vi "Read XML_Parse Read Data.vi"(6 "Close Ref?":bool=TRUE, 8 "error in (no error)":errorcluster, 11 ".NET Refnum in":refnum<k24>) -> (0 "error out":errorcluster, 2 ".NET Refnum out":refnum<k24>, 3 "Channels":T1[](array[typedef]))   [LabVIEW 2017]
uses:
  XML_Channel.ctl
  XML_Label.ctl
  XML_Parameter.ctl
  D:/Ballard-Arinc-429-Custom-Device/Source/System Explorer/SubVIs/Parse Parameters File/Parameters_Arinc429_XML_Tools.dll
  Ballard-Arinc-429-Custom-Device/Source/System Explorer/SubVIs/Parse Parameters File/Parameters_Arinc429_XML_Tools.dll
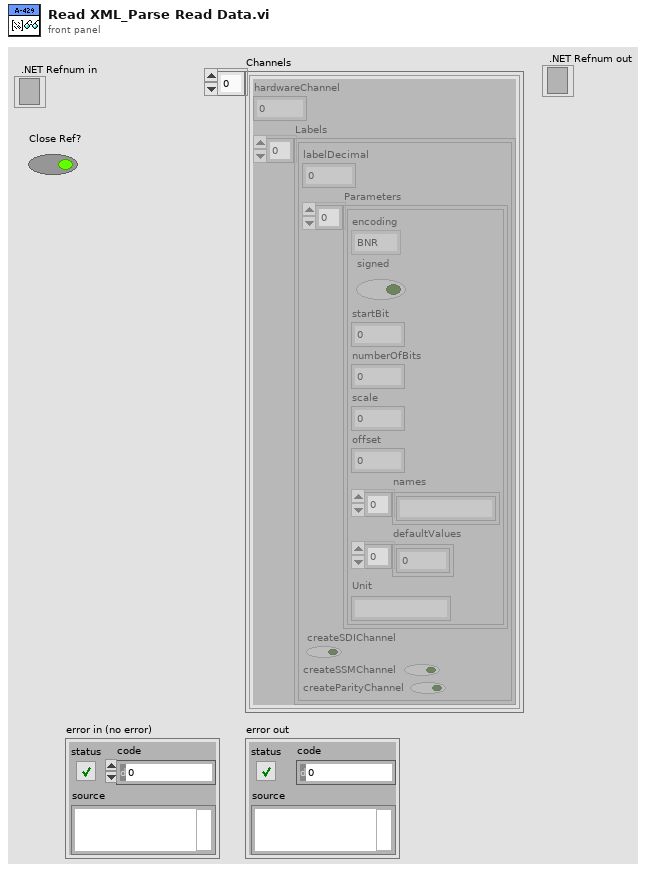
[diagram p1: front panel]
types:
  T1 = typedef "XML_Channel.ctl" = cluster{"hardwareChannel":i32, "Labels":T2[]}
  T2 = typedef "XML_Label.ctl" = cluster{"labelDecimal":i32, "Parameters":T3[], "createSDIChannel":bool, "createSSMChannel":bool, "createParityChannel":bool}
  T3 = typedef "XML_Parameter.ctl" = cluster{"encoding":enum16{"BNR", "BCD", "Discrete"}, "signed":bool, "startBit":i32, "numberOfBits":i32, "scale":dbl, "offset":dbl, "names":string[], "defaultValues":dbl[], "Unit":string}
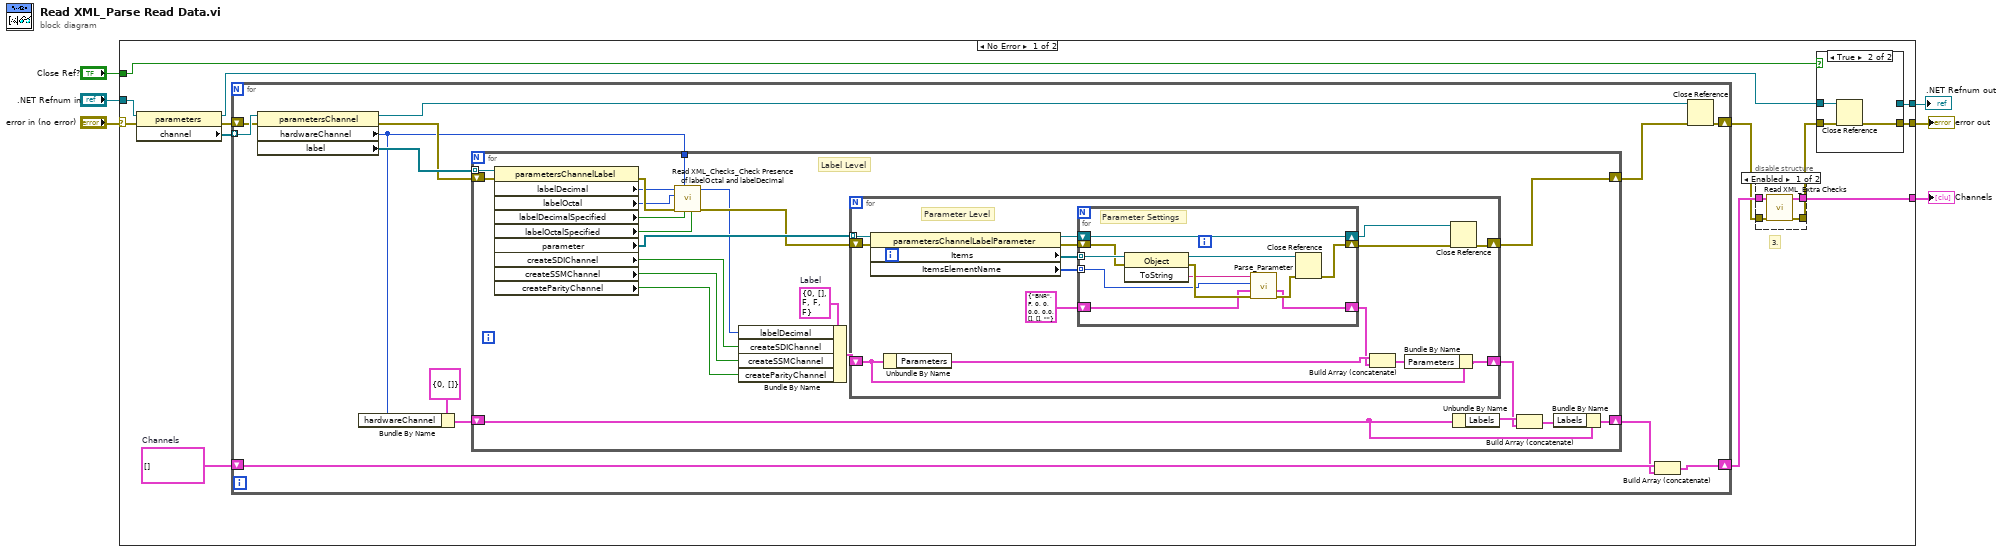
[diagram p0: block diagram]
diagram:
  n1 = case shown="No Error" "error in (no error)" {
    selector: "error in (no error)" -> [w9 w92]
    tunnel: [w17 _] -> w6
    tunnel: ".NET Refnum in" -> [w11 _]
    tunnel: [w10 w92] -> w4
    tunnel: "Close Ref?" -> [w8 _]
    tunnel: [w7 _] -> w1
    frame No Error {
      w18 = T1[] []  # Channels
      # "3."
      n2 = property class="parameters"(reference=w11, error in=w9) -> (reference out=w13:refnum<k24>, error out=w14:errorcluster, "channel"=w12:refnum<k24>[])
      n3 = for {
        tunnel: w12 -> [w43] mode=indexing
        shift-right: [w40] -> w15
        shift-left: w14 -> [w42]
        shift-right: [w33] -> w19
        shift-left: w18 -> [w34]
        n4 = property class="parametersChannel"(reference=w43, error in=w42) -> (reference out=w41:refnum<k24>, error out=w38:errorcluster, "hardwareChannel"=w31:i32, "label"=w39:refnum<k24>[])
        n5 = Bundle By Name(cluster=T1 {"hardwareChannel"=0, "Labels"=[]} ("Channel"), "hardwareChannel"=w31) -> (w35:T1)
        n6 = for {
          tunnel: w39 -> [w65] mode=indexing
          shift-right: [w62] -> w37
          shift-left: w38 -> [w64]
          shift-right: [w55] -> w32
          shift-left: w35 -> [w57]
          tunnel: w31 -> [w44]
          w61 = T2 {"labelDecimal"=0, "Parameters"=[], "createSDIChannel"=FALSE, "createSSMChannel"=FALSE, "createParityChannel"=FALSE}  # Label
          # "Label Level"
          n7 = property class="parametersChannelLabel"(reference=w65, error in=w64) -> (error out=w51:errorcluster, "labelDecimal"=w48:i32, "labelOctal"=w47:i32, "labelDecimalSpecified"=w46:bool, "labelOctalSpecified"=w45:bool, "parameter"=w63:refnum<k24>[], "createSDIChannel"=w54:bool, "createSSMChannel"=w53:bool, "createParityChannel"=w52:bool)  [unwired: 1 out]
          n8 = call "Read XML_Checks_Check Presence of labelOctal and labelDecimal.vi"("labelOctalSpecified"=w45, "labelDecimalSpecified"=w46, "hardwareChannel"=w44, "error in (no error)"=w51, "labelOctal"=w47, "labelDecimal"=w48) -> ("error out"=w50:errorcluster, "labelDecimal"=w49:i32)  [unwired: 4 in]
          n9 = Bundle By Name(cluster=w61, "labelDecimal"=w49, "createSDIChannel"=w54, "createSSMChannel"=w53, "createParityChannel"=w52) -> (w60:T2)
          n10 = for {
            tunnel: w63 -> [w79] mode=indexing
            shift-right: [w74] -> w62
            shift-left: w50 -> [w80]
            shift-right: [w69] -> w58
            shift-left: w60 -> [w70]
            # "Parameter Level"
            n11 = property class="parametersChannelLabelParameter"(reference=w79, error in=w80) -> (reference out=w78:refnum<k24>, error out=w77:errorcluster, "Items"=w73:refnum<k24>[], "ItemsElementName"=w72:i32[])
            n12 = Unbundle By Name(w70) -> ("Parameters"=w68:T3[])
            n13 = for {
              shift-right: [w90] -> w76
              shift-left: w77 -> [w88]
              shift-right: [w91] -> w75
              shift-left: w78 -> [w91]
              tunnel: w73 -> [w89] mode=indexing
              tunnel: w72 -> [w81] mode=indexing
              shift-right: [w82] -> w66
              shift-left: T3 {"encoding"=enum."BNR", "signed"=FALSE, "startBit"=0, "numberOfBits"=0, "scale"=0.0, "offset"=0.0, "names"=[], "defaultValues"=[], "Unit"=""} ("Parameter") -> [w83]
              # "Parameter Settings"
              n14 = invoke class="Object" method="ToString"(reference=w89, error in=w88) -> (reference out=w87:refnum<k24>, error out=w86:errorcluster, "ToString"=w84:string)  [unwired: 1 in]
              n15 = call "Parse_Parameter.vi"("error in (no error)"=w86, "Parameter In"=w83, "ItemName"=w81, "Value (String)"=w84) -> ("error out"=w85:errorcluster, "Parameter Out"=w82:T3)  [unwired: 6 in]
              n16 = Close Reference(reference=w87, error in (no error)=w85) -> (error out=w90:errorcluster)
            }
            n17 = Build Array (concatenate)(w68, w66) -> (w67:T3[])
            n18 = Bundle By Name(cluster=w70, "Parameters"=w67) -> (w69:T2)
            n19 = Close Reference(reference=w75, error in (no error)=w76) -> (error out=w74:errorcluster)
          }
          n20 = Unbundle By Name(w57) -> ("Labels"=w59:T2[])
          n21 = Build Array (concatenate)(w59, w58) -> (w56:T2[])
          n22 = Bundle By Name(cluster=w57, "Labels"=w56) -> (w55:T1)
        }
        n23 = Build Array (concatenate)(w34, w32) -> (w33:T1[])
        n24 = Close Reference(reference=w41, error in (no error)=w37) -> (error out=w40:errorcluster)
      }
      n25 = disable-structure shown="Enabled" {
        disable-tunnel: w15 -> [w28 w30]
        disable-tunnel: [w27 w30] -> w16
        disable-tunnel: [w26 w29] -> w17
        disable-tunnel: w19 -> [w25 w29]
        frame Enabled {
          n26 = call "Read XML_Extra Checks.vi"("error in (no error)"=w28, "Channels In"=w25) -> ("error out"=w27:errorcluster, "Channels Out"=w26:T1[])  [unwired: 8 in]
        }
        frame Disabled {
        }
      }
      n27 = case shown="True" w8 {
        tunnel: w16 -> [w21 w24]
        tunnel: w13 -> [w20 w23]
        tunnel: [w21 w22] -> w10
        tunnel: [w20 _] -> w7
        frame False {
        }
        frame True {
          n28 = Close Reference(reference=w23, error in (no error)=w24) -> (error out=w22:errorcluster)
        }
      }
    }
    frame Error {
    }
  }
  "Channels" <- w6
  "error out" <- w4
  ".NET Refnum out" <- w1
